vi "GetType.vi"(8 "error in (no error)":errorcluster, 11 "Acknowledge Fault Msg":refnum<class "Acknowledge Fault Msg.lvclass">) -> (0 "error out":errorcluster, 2 "Data Sample":variant, 3 "Acknowledge Fault Msg":refnum<class "Acknowledge Fault Msg.lvclass">)   [LabVIEW 2016, in "KIT-QVA.lvlib" / "Acknowledge Fault Msg.lvclass"]
doc: "This VI delivers a sample of the data type format the message expects."
uses:
  Acknowledge Fault Msg.lvclass
  Acknowledge Fault Msg.lvclass/Acknowledge Fault Msg.ctl
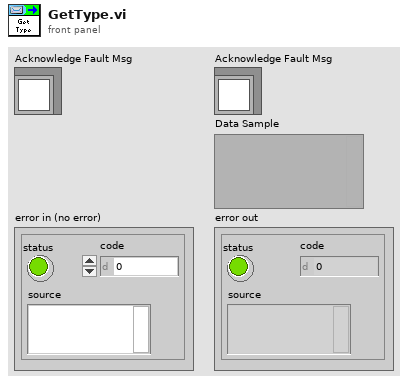
[diagram p1: front panel]
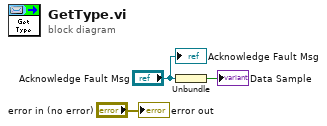
[diagram p0: block diagram]
diagram:
  n1 = Unbundle("Acknowledge Fault Msg") -> (→"Data Sample":bool)
  "error out" <- "error in (no error)"
  "Acknowledge Fault Msg" <- "Acknowledge Fault Msg"
